vi "Read ImageSave Message.vi"(8 "error in":errorcluster) -> (0 "error out":errorcluster, 2 "Message Received Parameters":variant, 3 "Message Received String":string, 5 "Message Recieved?":bool)   [LabVIEW 2012]
uses:
  MsgQ Loops enum.ctl
  Common/Interloop MessageQ/Message que instance modes enum.ctl
  Main MsgQ.lvlib
  Common/Interloop MessageQ/Interloop MessageQ.lvlib
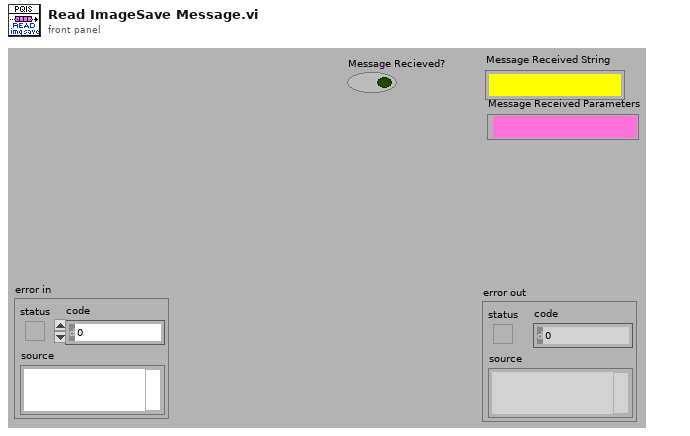
[diagram p1: front panel]
types:
  T1 = typedef "Interloop MessageQ.lvlib/Message que instance modes enum.ctl" = enum16{"Initialize", "Broadcast Message", "Send Message", "Read Message", "Kill"}
  T2 = typedef "Main MsgQ.lvlib/MsgQ Loops enum.ctl" = enum16{"User Interface", "File IO", "DIO", "Camera 1", "Camera 2", "Camera 3", "Camera 4", "Analysis", "Keyboard"}
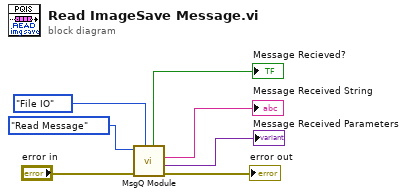
[diagram p0: block diagram]
diagram:
  n1 = call "MsgQ Module.vi"("MsgQ enum"=MsgQ_Loops_enum."File IO", "error in (no error)"="error in", "Mode"=Message_que_instance_modes_enum."Read Message") -> ("error out"=→"error out":errorcluster, "Message Received Parameters"=→"Message Received Parameters":variant, "Message Received String"=→"Message Received String":string, "Message Recieved?"=→"Message Recieved?":bool)  [unwired: 2 in, 3 out]
